vi "EffectivePowerTest.vi"() -> ()   [LabVIEW 2016]
uses:
  EffectivePowerState.ctl
  <vilib>/Platform/TimedLoop/XDataNode/timing_clust.ctl
  <vilib>/Platform/TimedLoop/XDataNode/nitl_modes.ctl
  <vilib>/Platform/TimedLoop/XDataNode/wakeup.ctl
  <vilib>/rvi/Emulation/niFpgaGetClockAttributes.vi
  <vilib>/rvi/Emulation/niFpgaSctlEmulationGetInTimedLoop.vi
  <vilib>/rvi/Emulation/niFpgaEmulationReportErrorSimple.vi
  <vilib>/rvi/eio/common/nirviEmuTemplateMethod_errors.vi
  <vilib>/rvi/Emulation/niFpgaCriticalErrorInLSC.vi
  <vilib>/eio/EIONode/EIONode.xnode
  <vilib>/platform/TimedLoop/XDataNode/XDataNode.xnode
  <vilib>/Platform/TimedLoop/XDataNode/XDNodeRunTimeDep.lvlib
panel:
  in  "Step Times (bits":i16[](array[numeric])=[0, 0, 0]
  in  "AOM Volt (bits)":u16[](array[numeric])=[0, 0, 0] max=2500 step=25
  in  "End Program 2":bool
  in  "End Program":bool
  # "Voltage Calibration\nThe myRIO attempts to give the following output voltages at these bit values, but doesn't provide enough current at 50 Ohms to achieve it.\n819=1V\n1638=2V\n2457=3V\n\nThese numbers for the voltages sent out from the AO channels  (IN0-IN3 in this vi) are in bits and must be calibrated to your coupling impedance at the OUT of the multiplexer.  Here's what I got in my case.\nVoltage output at 50 Ohms\nIN0 and IN3 MXP (A and B conectors)\n400->0.22V\n800->0.43V\n1200->0.64V\n1600->0.85V\n2000->1.06V\n\nVoltage output at 50 Ohms\nIN1 and IN2 MSP (C connector)\n100->0.21V\n200->0.42V\n300->0.63V\n400->0.84V\n500->1.04V\n\n25 ns/bit at 40MHz SCTL\n12.5 ns/bit at 80MHz SCTL"
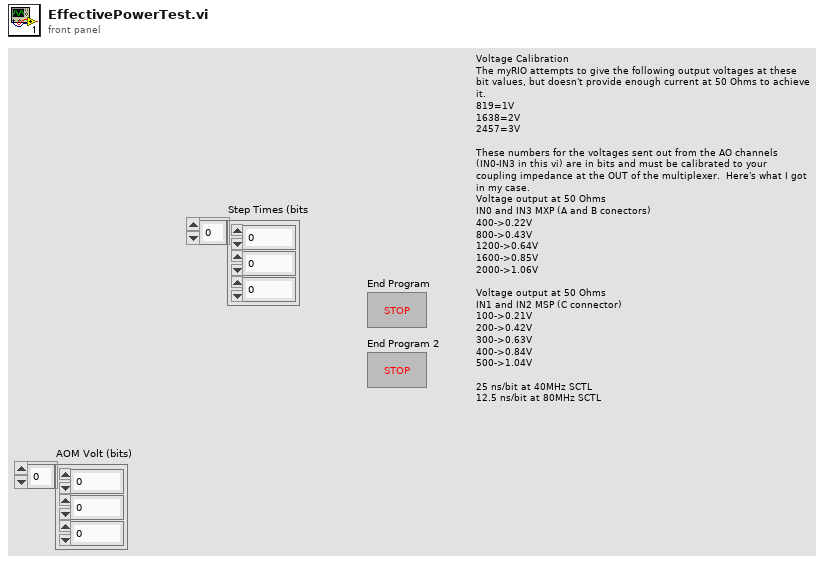
[diagram p1: front panel]
types:
  T1 = typedef "EffectivePowerState.ctl" = enum16{"Step 1", "Step 2", "Step 3"}
  T2 = typedef "XDNodeRunTimeDep.lvlib/timing_clust.ctl" = cluster{"Expected End [f-1]":u64, "Actual End [f-1]":u64, "Finished Late? [f-1]":bool, "Expected End [i-1]":u64, "Actual End [i-1]":u64, "Finished Late? [i-1]":bool, "Expected Start [i]":u64, "Actual Start [i]":u64, "Expected Start [f]":u64, "Actual Start [f]":u64, "Source Name":string, "Structure Name":string, "Period":i64, "Deadline":i64, "Offset":i64, "Start":i64, "Priority":i32, "Timeout":i32, "Mode":T3, "Wakeup Reason":T4, "Error":errorcluster, "Source Type":string, "Secondary Source Type":string, "Global End Time":u64, "Global Start Time":u64, "Frame Duration":u64, "Iteration Duration":u64, "Assigned CPU":i32, "I/O Scan Engine Mode":u32}
  T3 = typedef "XDNodeRunTimeDep.lvlib/nitl_modes.ctl" = enum32{"No Change", "Process missed periods, maintain original phase", "Discard missed periods, maintain original phase", "Process missed periods, ignore original phase", "Discard missed periods, ignore original phase"}
  T4 = typedef "XDNodeRunTimeDep.lvlib/wakeup.ctl" = enum32{"Normal", "Aborted", "Asynchronous wakeup", "Timing source error", "Timed loop error", "Timeout"}
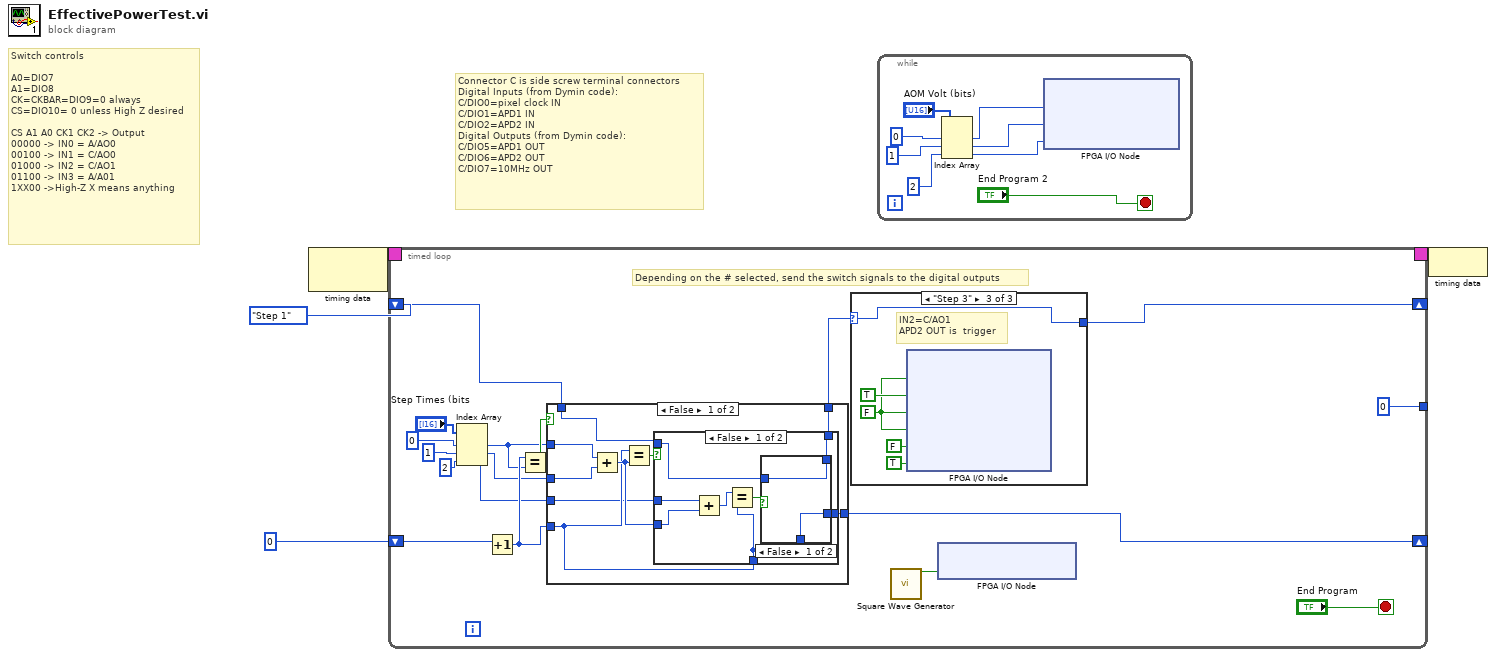
[diagram p0: block diagram]
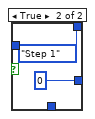
[diagram p2: hidden frame]
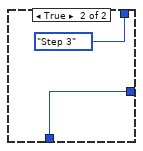
[diagram p3: hidden frame]
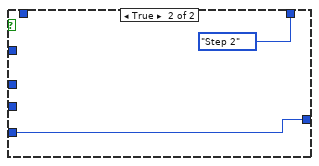
[diagram p4: hidden frame]
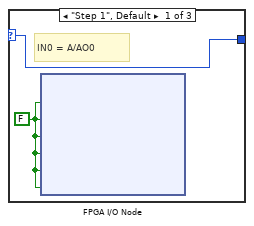
[diagram p5: hidden frame]
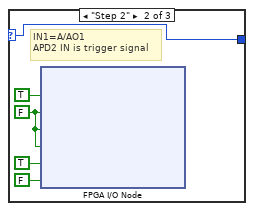
[diagram p6: hidden frame]
diagram:
  # "Switch controls\n\nA0=DIO7\nA1=DIO8\nCK=CKBAR=DIO9=0 always\nCS=DIO10= 0 unless High Z desired\n\nCS A1 A0 CK1 CK2 -> Output\n00000 -> IN0 = A/AO0\n00100 -> IN1 = C/AO0\n01000 -> IN2 = C/AO1\n01100 -> IN3 = A/A01\n1XX00 ->High-Z X means anything"
  # "Connector C is side screw terminal connectors\nDigital Inputs (from Dymin code):\nC/DIO0=pixel clock IN\nC/DIO1=APD1 IN\nC/DIO2=APD2 IN\nDigital Outputs (from Dymin code):\nC/DIO5=APD1 OUT\nC/DIO6=APD2 OUT\nC/DIO7=10MHz OUT"
  n1 = node-c288() -> (w4:T2)  [unwired: 1 in]
  n2 = timed-loop {
    tunnel: [i8 0 ("switch value of x")] -> _
    timing: w4 -> [_]
    timing-out: [_] -> w3
    shift-right: [w18] -> _
    shift-left: i16 0 -> [w20]
    shift-right: [w12] -> _
    shift-left: EffectivePowerState."Step 1" ("Numeric") -> [w13]
    stop <- "End Program" stop-if-true
    # "Depending on the # selected, send the switch signals to the digital outputs"
    n3 = Index Array(array="Step Times (bits", index #1=0 ("index"), index #2=1 ("index"), index #3=2 ("index")) -> (element #1=w9:i16, element #2=w6:i16, element #3=w5:i16)
    n4 = Increment(x=w20) -> (x+1=w15:i16)
    n5 = Equal?(x=w15, y=w9) -> (x = y?=w19:bool)
    n6 = case shown="False" w19 {
      tunnel: w9 -> [w30 _]
      tunnel: w15 -> [w27 w46]
      tunnel: [w25 EffectivePowerState."Step 2" ("Numeric")] -> w14
      tunnel: [w26 w46] -> w18
      tunnel: w13 -> [w24 _]
      tunnel: w6 -> [w23 _]
      tunnel: w5 -> [w22 _]
      frame False {
        n7 = Add(x=w30, y=w23) -> (x+y=w28:i16)
        n8 = Equal?(x=w27, y=w28) -> (x = y?=w29:bool)
        n9 = case shown="False" w29 {
          tunnel: [w36 EffectivePowerState."Step 3" ("Numeric")] -> w25
          tunnel: w28 -> [w34 _]
          tunnel: w27 -> [w32 w44]
          tunnel: [w37 w44] -> w26
          tunnel: w24 -> [w35 _]
          tunnel: w22 -> [w31 _]
          frame False {
            n10 = Add(x=w31, y=w34) -> (x+y=w33:i16)
            n11 = Equal?(x=w33, y=w32) -> (x = y?=w38:bool)
            n12 = case shown="False" w38 {
              tunnel: [w40 i16 0] -> w37
              tunnel: w32 -> [w40 _]
              tunnel: [w39 EffectivePowerState."Step 1" ("Numeric")] -> w36
              tunnel: w35 -> [w39 _]
              frame False {
              }
              frame True {
              }
            }
          }
          frame True {
          }
        }
      }
      frame True {
      }
    }
    n13 = case shown="\"Step 3\"" w14 {
      selector: w14 -> [w47 w49 w54]
      tunnel: [w47 w49 w54] -> w12
      frame "Step 1", Default {
        w48 = FALSE ("ConnectorA/DIO0")
        # "IN0 = A/AO0"
        n14 = xnode "FPGA I/O Node"("ConnectorA/DIO7"=w48, "ConnectorA/DIO8"=w48, "ConnectorA/DIO9"=w48, "ConnectorA/DIO10"=w48, "ConnectorC/DIO2"=w48, "ConnectorC/DIO6"=w48) -> ()  [unwired: 6 in, 6 out]
      }
      frame "Step 2" {
        w51 = FALSE ("ConnectorA/DIO1")
        # "IN1=A/AO1\nAPD2 IN is trigger signal"
        n15 = xnode "FPGA I/O Node"("ConnectorA/DIO7"=TRUE, "ConnectorA/DIO8"=w51, "ConnectorA/DIO9"=w51, "ConnectorA/DIO10"=w51, "ConnectorC/DIO2"=TRUE ("ConnectorA/DIO5"), "ConnectorC/DIO6"=FALSE ("ConnectorA/DIO5")) -> ()  [unwired: 6 in, 6 out]
      }
      frame "Step 3" {
        w57 = FALSE
        # "IN2=C/AO1\nAPD2 OUT is  trigger"
        n16 = xnode "FPGA I/O Node"("ConnectorA/DIO7"=w57, "ConnectorA/DIO8"=TRUE ("ConnectorA/DIO3"), "ConnectorA/DIO9"=w57, "ConnectorA/DIO10"=w57, "ConnectorC/DIO2"=FALSE ("ConnectorA/DIO2"), "ConnectorC/DIO6"=TRUE) -> ()  [unwired: 6 in, 6 out]
      }
    }
    n17 = call "Square Wave Generator"() -> ("square wave out"=w16:bool)  [unwired: 15 in]
    n18 = xnode "FPGA I/O Node"("ConnectorC/DIO7"=w16) -> ()  [unwired: 1 in, 1 out]
  }
  n19 = while {
    stop <- "End Program 2" stop-if-true
    n20 = Index Array(array="AOM Volt (bits)", index #1=0 ("index"), index #2=1 ("index"), index #3=2 ("index")) -> (element #1=w63:u16, element #2=w62:u16, element #3=w61:u16)
    n21 = xnode "FPGA I/O Node"("ConnectorA/AO0"=w63, "ConnectorC/AO0"=w62, "ConnectorC/AO1"=w61) -> ()  [unwired: 3 in, 3 out]
  }
  n22 = node-c288(w3) -> ()
